vi "DN4_EventCounting_GetValue_Ex.vi"(3 "error in (no error)":errorcluster, 5 "Task ID":u32) -> (0 "error out":errorcluster, 1 "counts":u32[](array[numeric]), 2 "Task ID":u32)   [LabVIEW 2009]
uses:
  Windows/System32/AdvLvDaq.dll
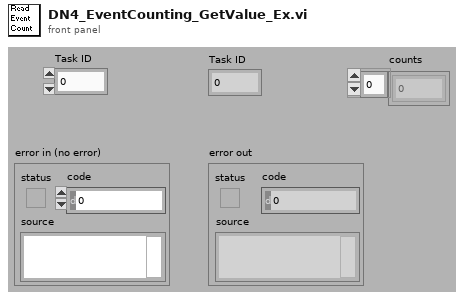
[diagram p1: front panel]
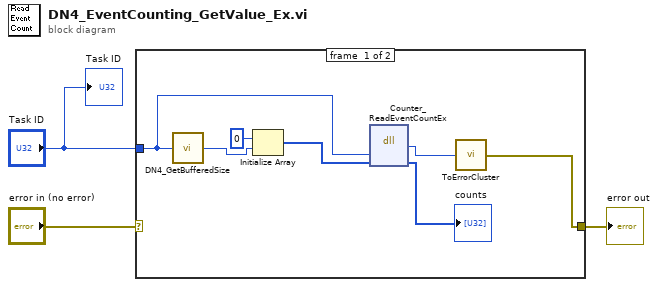
[diagram p0: block diagram]
diagram:
  n1 = case shown="Error" "error in (no error)" {
    selector: "error in (no error)" -> [_ w11]
    tunnel: [w5 w11] -> w2
    tunnel: "Task ID" -> [w7 _]
    frame #0 {
      n2 = call <userlib>:"DN4_GetBufferedSize.vi"("Task ID"=w7) -> ("return type"=w9:i32)
      n3 = Initialize Array(0 ("element"), w9) -> (w8:i32[])
      n4 = dll-call lib="C:/Windows/System32/AdvLvDaq.dll" fn="Counter_ReadEventCountEx"("taskId"=w7, "count"=w8) -> ("return type"=w6:i32, "count"=→"counts":i32[])  [unwired: 4 in, 2 out]
      n5 = call <userlib>:"ToErrorCluster.vi"("error code"=w6) -> ("error out"=w5:errorcluster)
    }
    frame #1 {
    }
  }
  "error out" <- w2
  "Task ID" <- "Task ID"
